vi "SA Cond - Apply TDF.vi"(0 "Signals IN":waveform(dbl)[](array[waveform]), 6 "Anotate Signal Name":bool=TRUE, 7 "TDF Parameters":T1 {"stopband attenuation (dB)" format="%.2f"; "passband ripple (dB)" format="%.2f"; "HP cutoff freq" format="%#.3f"; "LP cutoff freq" format="%#.3f"}) -> (14 "Signals OUT":waveform(dbl)[](array[waveform]))   [LabVIEW 2022 SP3, in "GSwFormDSP.lvclass"]
uses:
  GSwFormDSP.lvclass
  TDF Parameters.ctl
  <vilib>/Analysis/baseanly.llb/IIR Cascade Filter (DBL).vi
  <vilib>/Analysis/NI_AALBase.lvlib
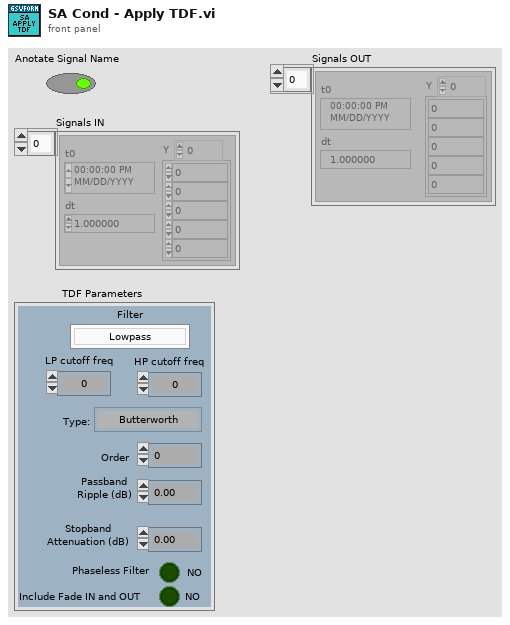
[diagram p1: front panel]
types:
  T1 = typedef "GSwFormDSP.lvclass/TDF Parameters.ctl" = cluster{"Filter":enum32{"Lowpass", "Highpass", "Bandpass", "Bandstop"}, "Type:":enum16{"Butterworth", "Chebyshev", "Inv Chebyshev", "Elliptic", "Bessel"}, "LP cutoff freq":dbl, "HP cutoff freq":dbl, "Order":i32, "passband ripple (dB)":dbl, "stopband attenuation (dB)":dbl, "Phaseless Filter":bool, "Include Fade IN and OUT":bool}
  T2 = enum16{"Butterworth", "Chebyshev", "Inv Chebyshev", "Elliptic", "Bessel"}
  T3 = enum32{"Lowpass", "Highpass", "Bandpass", "Bandstop"}
  T4 = cluster{"filter structure":enum32{"IIR 2nd Order", "IIR 4th Order"}, "Reverse Coefficients":dbl[], "Forward Coefficients":dbl[]}
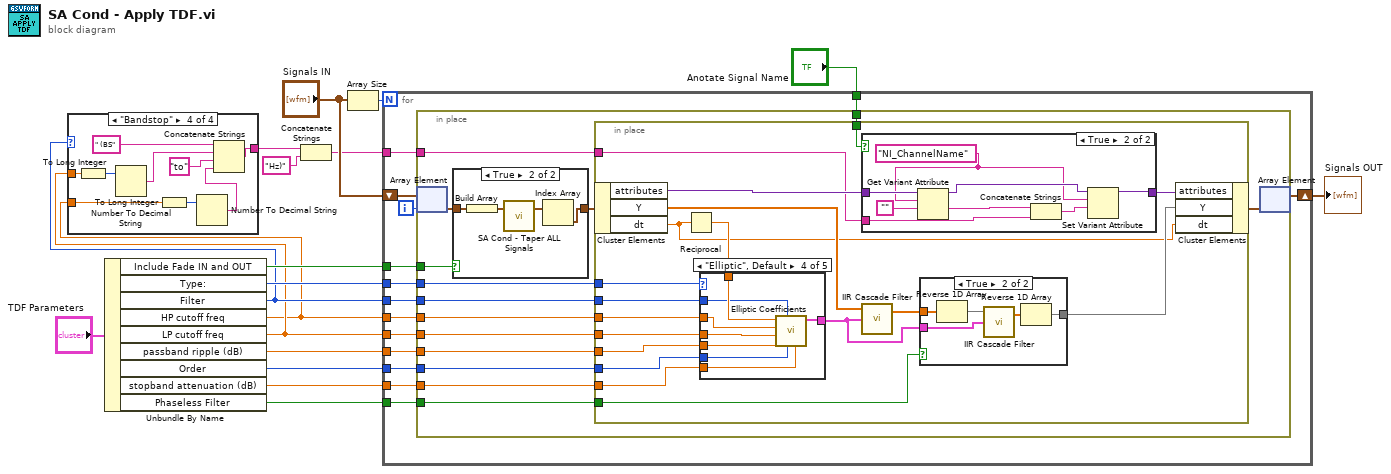
[diagram p0: block diagram]
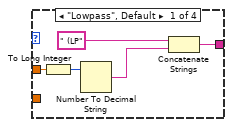
[diagram p2: hidden frame]
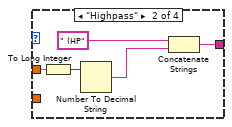
[diagram p3: hidden frame]
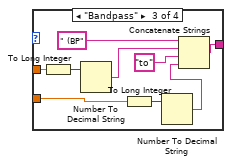
[diagram p4: hidden frame]
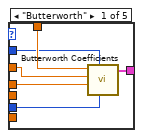
[diagram p8: hidden frame]
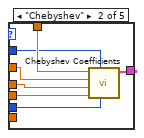
[diagram p9: hidden frame]
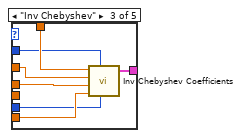
[diagram p10: hidden frame]
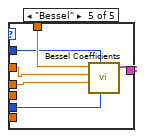
[diagram p11: hidden frame]
diagram:
  n1 = Unbundle By Name("TDF Parameters") -> ("Include Fade IN and OUT"=w17:bool, "Type:"=w9:T2, "Filter"=w6:T3, "HP cutoff freq"=w1:dbl, "LP cutoff freq"=w5:dbl, "passband ripple (dB)"=w10:dbl, "Order"=w11:i32, "stopband attenuation (dB)"=w12:dbl, "Phaseless Filter"=w8:bool)
  n2 = case shown="\"Bandstop\"" w6 {
    tunnel: w5 -> [w22 w27 w36 w45]
    tunnel: [w18 w23 w32 w41] -> w3
    tunnel: w1 -> [_ _ w30 w39]
    frame "Lowpass", Default {
      n3 = To Long Integer(number=w22) -> (32bit integer=w21:i32)
      n4 = Number To Decimal String(number=w21) -> (decimal integer string=w20:string)  [unwired: 1 in]
      n5 = Concatenate Strings(" (LP", w20) -> (w18:string)
    }
    frame "Highpass" {
      n6 = To Long Integer(number=w27) -> (32bit integer=w26:i32)
      n7 = Number To Decimal String(number=w26) -> (decimal integer string=w25:string)  [unwired: 1 in]
      n8 = Concatenate Strings(" (HP", w25) -> (w23:string)
    }
    frame "Bandpass" {
      n9 = To Long Integer(number=w36) -> (32bit integer=w35:i32)
      n10 = Number To Decimal String(number=w35) -> (decimal integer string=w34:string)  [unwired: 1 in]
      n11 = To Long Integer(number=w30) -> (32bit integer=w31:i32)
      n12 = Number To Decimal String(number=w31) -> (decimal integer string=w29:string)  [unwired: 1 in]
      n13 = Concatenate Strings(" (BP", w34, "to", w29) -> (w32:string)
    }
    frame "Bandstop" {
      n14 = To Long Integer(number=w45) -> (32bit integer=w44:i32)
      n15 = Number To Decimal String(number=w44) -> (decimal integer string=w43:string)  [unwired: 1 in]
      n16 = To Long Integer(number=w39) -> (32bit integer=w40:i32)
      n17 = Number To Decimal String(number=w40) -> (decimal integer string=w38:string)  [unwired: 1 in]
      n18 = Concatenate Strings(" (BS", w43, "to", w38) -> (w41:string)
    }
  }
  n19 = Concatenate Strings(w3, "Hz)") -> (w2:string)
  n20 = Array Size(array="Signals IN") -> (size(s)=w7:i32)
  n21 = for {
    N: w7 -> [_]
    tunnel: w12 -> [w59]
    tunnel: w11 -> [w58]
    tunnel: w10 -> [w57]
    tunnel: w5 -> [w56]
    tunnel: w9 -> [w55]
    tunnel: w8 -> [w54]
    tunnel: w6 -> [w53]
    tunnel: w1 -> [w52]
    tunnel: "Anotate Signal Name" -> [w51]
    shift-right: [w48] -> w15
    shift-left: "Signals IN" -> [w50]
    tunnel: w2 -> [w47]
    tunnel: w17 -> [w46]
    i -> [w49]
    n22 = in-place {
      in-place-border: w59 -> [w73]
      in-place-border: w58 -> [w72]
      in-place-border: w57 -> [w71]
      in-place-border: w56 -> [w70]
      in-place-border: w55 -> [w69]
      in-place-border: w54 -> [w68]
      in-place-border: w53 -> [w67]
      in-place-border: w52 -> [w66]
      in-place-border: w51 -> [w65]
      in-place-border: w47 -> [w63]
      in-place-border: w46 -> [w62]
      n23 = in-place-array #1(w50, w49) -> (w60:waveform(dbl))
      n24 = case shown="True" w62 {
        tunnel: [w74 w76] -> w61
        tunnel: w60 -> [w74 w78]
        frame False {
        }
        frame True {
          n25 = Build Array(w78) -> (w75:waveform(dbl)[])
          n26 = call "SA Cond - Taper ALL Signals.vi"("wForm IN"=w75) -> ("wForm OUT"=w77:waveform(dbl)[])  [unwired: 17 in, 1 out]
          n27 = Index Array(array=w77) -> (element=w76:waveform(dbl))  [unwired: 1 in]
        }
      }
      n28 = in-place {
        in-place-border: w73 -> [w96]
        in-place-border: w72 -> [w95]
        in-place-border: w71 -> [w94]
        in-place-border: w70 -> [w93]
        in-place-border: w69 -> [w92]
        in-place-border: w68 -> [w91]
        in-place-border: w67 -> [w88]
        in-place-border: w66 -> [w87]
        in-place-border: w65 -> [w86]
        in-place-border: w63 -> [w79]
        n29 = in-place-cluster #2(w61) -> ("attributes"=w82:variant, "Y"=w84:dbl[], "dt"=w80:dbl)
        n30 = Reciprocal(x=w80) -> (1/x=w85:dbl)
        n31 = case shown="\"Elliptic\", Default" w92 {
          tunnel: w85 -> [w117 w124 w131 w139 w145]
          tunnel: w93 -> [w116 w123 w130 w138 w144]
          tunnel: w94 -> [_ w122 _ w137 _]
          tunnel: w95 -> [w115 w121 w128 w136 w143]
          tunnel: w96 -> [_ _ w129 w135 _]
          tunnel: [w114 w120 w127 w134 w142] -> w89
          tunnel: w88 -> [w113 w119 w126 w133 w141]
          tunnel: w87 -> [w112 w118 w125 w132 w140]
          frame "Butterworth" {
            n32 = call <vilib>:"Butterworth Coefficients.vi"("order"=w115, "filter type"=w113, "low cutoff freq: fl"=w116, "high cutoff freq: fh"=w112, "sampling freq: fs"=w117) -> ("IIR Filter Cluster"=w114:T4)  [unwired: 5 in, 1 out]
          }
          frame "Chebyshev" {
            n33 = call <vilib>:"Chebyshev Coefficients.vi"("order"=w121, "filter type"=w119, "ripple(dB)"=w122, "low cutoff freq: fl"=w123, "high cutoff freq: fh"=w118, "sampling freq: fs"=w124) -> ("IIR Filter Cluster"=w120:T4)  [unwired: 4 in, 1 out]
          }
          frame "Inv Chebyshev" {
            n34 = call <vilib>:"Inv Chebyshev Coefficients.vi"("order"=w128, "filter type"=w126, "attenuation (dB)"=w129, "low cutoff freq: fl"=w130, "high cutoff freq: fh"=w125, "sampling freq: fs"=w131) -> ("IIR Filter Cluster"=w127:T4)  [unwired: 4 in, 1 out]
          }
          frame "Elliptic", Default {
            n35 = call <vilib>:"Elliptic Coefficients.vi"("stopband attenuation (dB)"=w135, "order"=w136, "filter type"=w133, "passband ripple (dB)"=w137, "low cutoff freq: fl"=w138, "high cutoff freq: fh"=w132, "sampling freq: fs"=w139) -> ("IIR Filter Cluster"=w134:T4)  [unwired: 3 in, 1 out]
          }
          frame "Bessel" {
            n36 = call <vilib>:"Bessel Coefficients.vi"("order"=w143, "filter type"=w141, "low cutoff freq: fl"=w144, "high cutoff freq: fh"=w140, "sampling freq: fs"=w145) -> ("IIR Filter Cluster"=w142:T4)  [unwired: 5 in, 1 out]
          }
        }
        n37 = case shown="True" w86 {
          tunnel: [w97 w102] -> w83
          tunnel: w82 -> [w97 w105]
          tunnel: w79 -> [_ w98]
          frame False {
          }
          frame True {
            w99 = "NI_ChannelName" ("Att - wform Name")
            n38 = Get Variant Attribute(Variant=w105, name=w99, default value (empty Variant)="") -> (duplicate Variant=w101:variant, value=w103:string)  [unwired: 1 in, 2 out]
            n39 = Concatenate Strings(w103, w98) -> (w100:string)
            n40 = Set Variant Attribute(Variant=w101, name=w99, value=w100) -> (Variant out=w102:variant)  [unwired: 1 in, 2 out]
          }
        }
        n41 = call-poly <vilib>:"IIR Cascade Filter.vi"("IIR Filter Cluster"=w89, "X"=w84) -> ("Filtered X"=w90:dbl[])  [unwired: 1 in, 1 out]
        n42 = case shown="True" w91 {
          tunnel: w90 -> [w106 w111]
          tunnel: [w106 w107] -> w81
          tunnel: w89 -> [_ w109]
          frame False {
          }
          frame True {
            n43 = Reverse 1D Array(array=w111) -> (reversed array=w110:dbl[])
            n44 = call-poly <vilib>:"IIR Cascade Filter.vi"("IIR Filter Cluster"=w109, "X"=w110) -> ("Filtered X"=w108:dbl[])  [unwired: 1 in, 1 out]
            n45 = Reverse 1D Array(array=w108) -> (reversed array=w107:dbl[])
          }
        }
        n46 = in-place-cluster #2("attributes"=w83, "Y"=w81, "dt"=w80) -> (w64:waveform(dbl))
      }
      n47 = in-place-array #1(w64) -> (w48:waveform(dbl)[])  [unwired: 1 out]
    }
  }
  "Signals OUT" <- w15
